vi "Initialize.vi"(8 "error in (no error)":errorcluster, 11 "VISA resource name":string) -> (0 "error out":errorcluster, 3 "reference out":refnum<k24>)   [LabVIEW 2017, in "piezojena NV40Single.lvlib"]
doc: "Open the device denoted by <b>VISA resource name</b> and initialize communication.\nAfter running this VI, <b>reference out</b> should be closed even if <b>error out</b> is an error."
uses:
  piezojena NV40Single.lvlib
  C:/Users/Spenser Burrows/Desktop/Work/Labview software for spectrometer/PiezoStage_John/Piezojena.Protocols.Nv40Single.dll
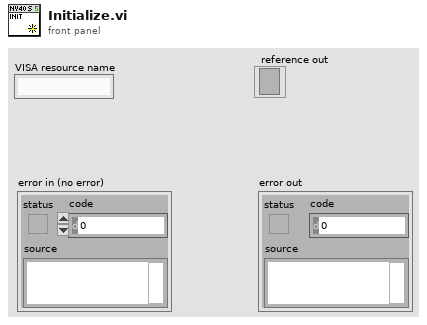
[diagram p1: front panel]
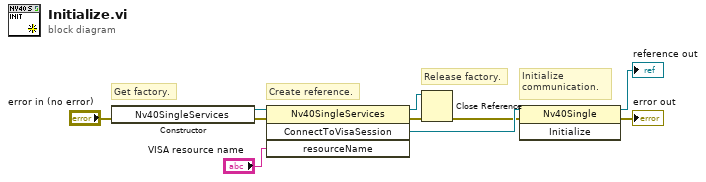
[diagram p0: block diagram]
diagram:
  # "Initialize\ncommunication."
  # "Release factory."
  # "Create reference."
  # "Get factory."
  n1 = constructor class="Nv40SingleServices"(error in="error in (no error)") -> (reference out=w10:refnum<k24>, error out=w9:errorcluster)  [unwired: 2 in, 1 out]
  n2 = invoke class="Nv40SingleServices" method="ConnectToVisaSession"(reference=w10, error in=w9, "resourceName"="VISA resource name") -> (reference out=w6:refnum<k24>, error out=w5:errorcluster, "ConnectToVisaSession"=w7:refnum<k24>)  [unwired: 1 in, 1 out]
  n3 = Close Reference(reference=w6, error in (no error)=w5) -> (error out=w4:errorcluster)
  n4 = invoke class="Nv40Single" method="Initialize"(reference=w7, error in=w4) -> (reference out=→"reference out":refnum<k24>, error out=→"error out":errorcluster)  [unwired: 1 in, 1 out]
